vi "RX OOB Test Cases.vi"() -> (0 "error out":errorcluster, 2 "status":string, 3 "pass":bool)   [LabVIEW 2021]
uses:
  OOB_Rx/ChanMngOOB_Rx.lvclass/ChanMngOOB_Rx.ctl
  <vilib>/CIF Foundation/CIF Out of Band Commands/CIFOutOfBand.lvclass/CIFOutOfBand.ctl
  OOB_Rx/Typedef/OOB ChnMng Commands.ctl
  OOB_Rx/Typedef/Channel Connection Data.ctl
  OOB_Rx/Typedef/Channel Fault Data.ctl
  OOB_Rx/Typedef/FIFO Publisher.ctl
  <vilib>/CIF Foundation/CIF Channels Core/ChannelCommon/typedef/New FIFO Instance Configuration.ctl
  OOB_Rx/Private/Command Settings.vi
  <vilib>/CIF Foundation/CIF Out of Band Commands/Accessors/Write Local OOB Data.vi
  <vilib>/CIF Foundation/CIF Out of Band Commands/Accessors/Read Local OOB Data.vi
  <vilib>/CIF Foundation/CIF Out of Band Commands/Queue Command.vi
  <vilib>/CIF Foundation/CIF Out of Band Commands/Utilities/Command to Bitwise Command.vi
  <vilib>/CIF Foundation/CIF Out of Band Commands/Read Commands.vi
  OOB_Rx/Private/Read Payload.vi
  OOB_Rx/ChanMngOOB_Rx.lvclass
  C:/Program Files/National Instruments/LabVIEW 2021/vi.lib/CIF Foundation/CIF Out of Band Commands/CIFOutOfBand.lvclass
  <vilib>/CIF Foundation/CIF Out of Band Commands/Init OOB.vi
  <vilib>/CIF Foundation/CIF Out of Band Commands/CIFOutOfBand.lvclass
  <vilib>/CIF Foundation/CIF Channels Core/ChannelCommon/ChannelCommon.lvlib
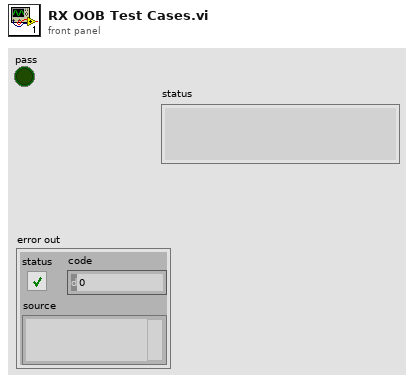
[diagram p1: front panel]
types:
  T1 = typedef "ChanMngOOB_Rx.lvclass/OOB ChnMng Commands.ctl" = enum8{"Connect Channel", "Force Channel", "Add FIFO Pub", "Remove FIFO Pub"}
  T2 = typedef "ChanMngOOB_Rx.lvclass/Channel Connection Data.ctl" = cluster{"Publisher Name":string, "Subscriber Name":string, "Connection Data":u8[]}
  T3 = typedef "ChanMngOOB_Rx.lvclass/Channel Fault Data.ctl" = cluster{"Channel Name":string, "Force Data":u8[], "Force Active":bool}
  T4 = typedef "ChanMngOOB_Rx.lvclass/FIFO Publisher.ctl" = cluster{"Publisher Name":string, "New FIFO Instance Config":T5}
  T5 = typedef "ChannelCommon.lvlib/New FIFO Instance Configuration.ctl" = cluster{"Primary":bool, "Backpressure":bool, "Message/FIFO Override":u32}
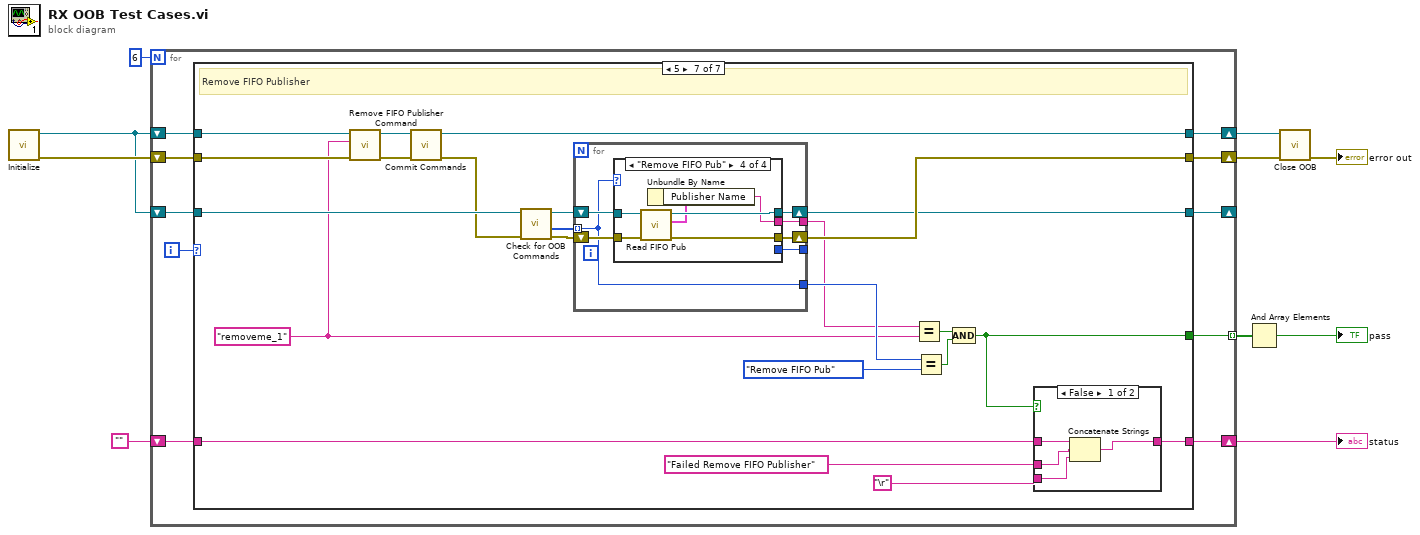
[diagram p0: block diagram]
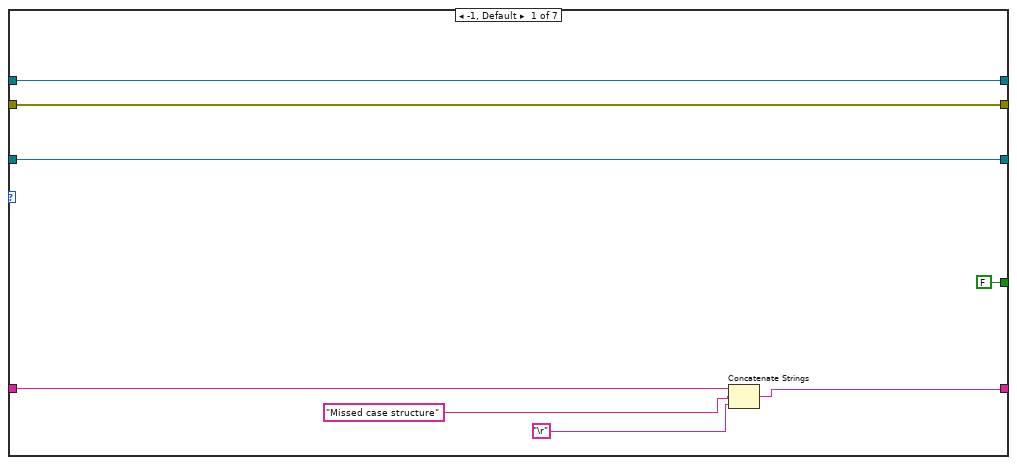
[diagram p2: hidden frame]
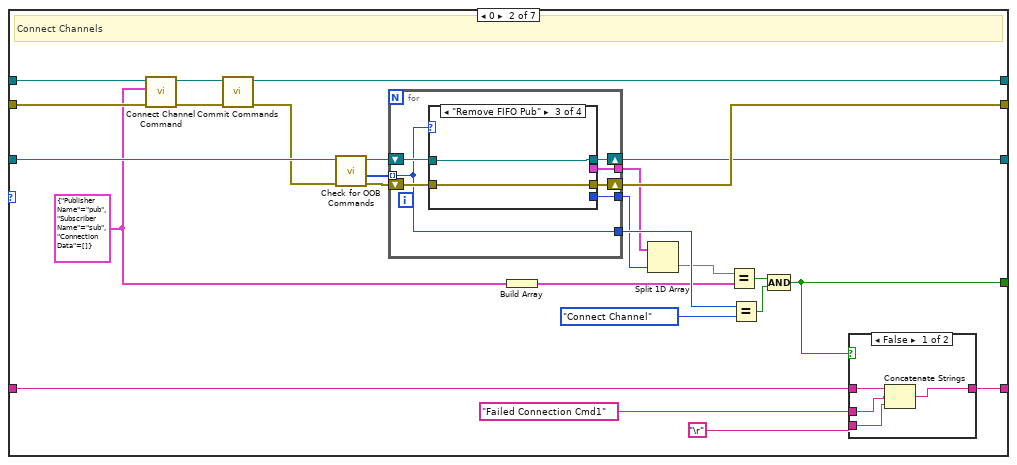
[diagram p3: hidden frame]
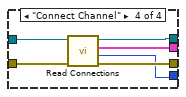
[diagram p6: hidden frame]
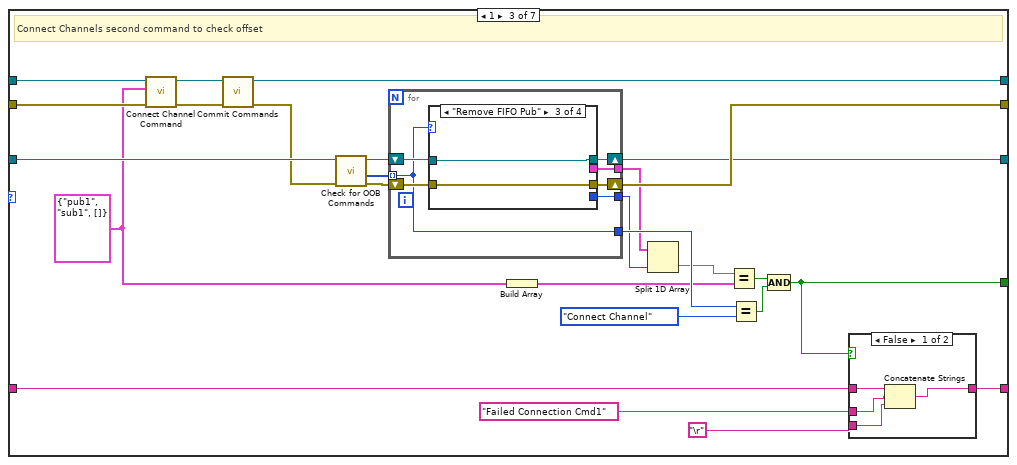
[diagram p8: hidden frame]
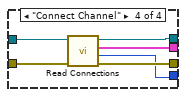
[diagram p11: hidden frame]
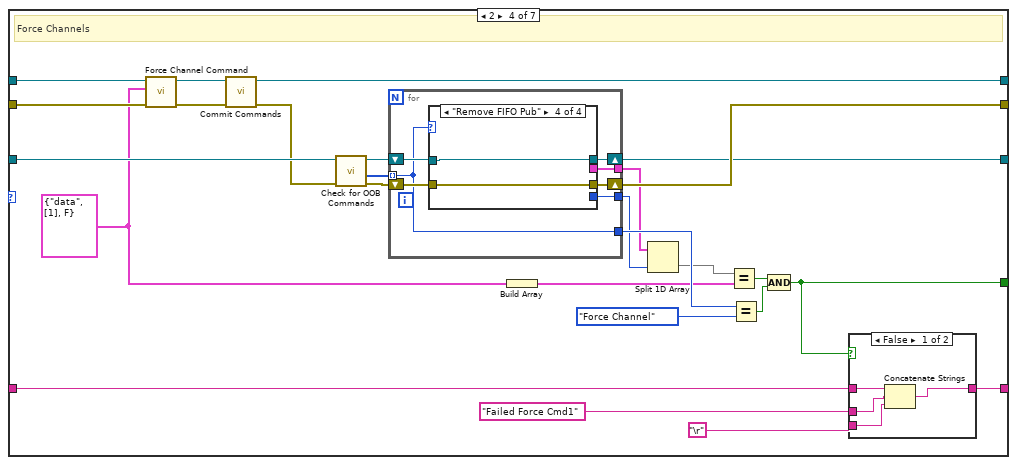
[diagram p13: hidden frame]
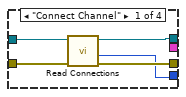
[diagram p14: hidden frame]
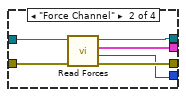
[diagram p15: hidden frame]
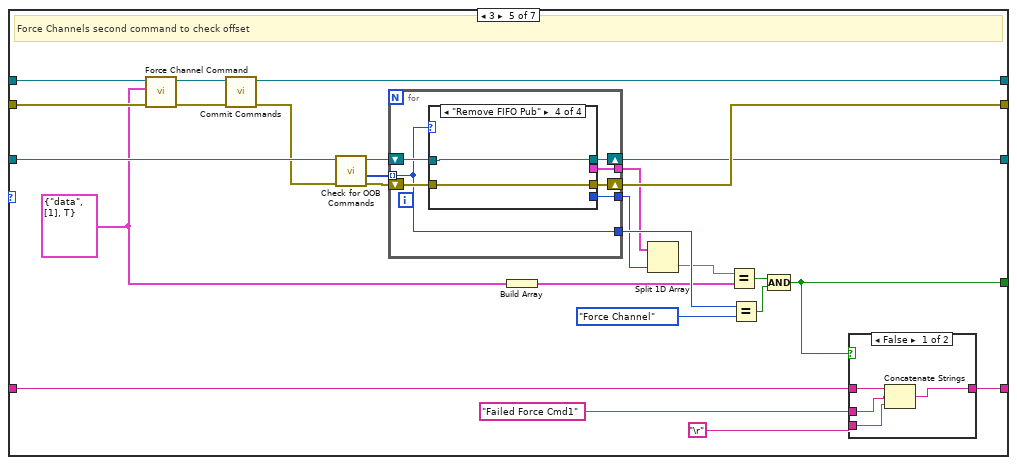
[diagram p18: hidden frame]
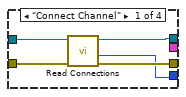
[diagram p19: hidden frame]
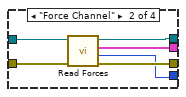
[diagram p20: hidden frame]
diagram:
  n1 = call "Initialize.vi"() -> ("error out"=w2:errorcluster, "CoreOOB_Rx out"=w1:refnum<class "ChanMngOOB_Rx.lvclass">)  [unwired: 10 in]
  n2 = for {
    N: 6 -> [_]
    tunnel: [w20] -> w8 mode=indexing
    shift-right: [w17] -> w9
    shift-left: w2 -> [w19]
    shift-right: [w15] -> w10
    shift-left: w1 -> [w18]
    shift-right: [w13] -> _
    shift-left: w1 -> [w14]
    shift-right: [w11] -> w5
    shift-left: "" -> [w12]
    i -> [w16]
    n3 = case shown="5" w16 {
      tunnel: [FALSE w33 w83 w135 w188 w243 w295] -> w20
      tunnel: w19 -> [w26 w41 w91 w141 w194 w238 w289]
      tunnel: w18 -> [w28 w42 w92 w142 w195 w240 w291]
      tunnel: [w26 w54 w104 w154 w207 w257 w309] -> w17
      tunnel: [w28 w29 w79 w129 w182 w241 w293] -> w15
      tunnel: w14 -> [w27 w48 w98 w148 w201 w251 w303]
      tunnel: [w27 w53 w103 w153 w206 w256 w308] -> w13
      tunnel: w12 -> [w23 w52 w102 w152 w205 w255 w307]
      tunnel: [w22 w51 w101 w151 w204 w254 w306] -> w11
      frame -1, Default {
        n4 = Concatenate Strings(w23, "Missed case structure", "\r") -> (w22:string)
      }
      frame 0 {
        w37 = T2 {"Publisher Name"="pub", "Subscriber Name"="sub", "Connection Data"=[]} ("Channel Connection Data")
        # "Connect Channels"
        n5 = call "Connect Channel Command.vi"("error in"=w41, "Channel Connection Data"=w37, "CoreOOB_Rx in"=w42) -> ("error out"=w31:errorcluster, "CoreOOB_Rx out"=w32:refnum<class "ChanMngOOB_Rx.lvclass">)  [unwired: 7 in]
        n6 = call <vilib>:"Commit Commands.vi"("error in"=w31, "OOB in"=w32) -> ("error out"=w30:errorcluster, "OOB out"=w29:refnum<class "ChanMngOOB_Rx.lvclass">)  [unwired: 8 in]
        n7 = call "Check for OOB Commands.vi"("error in (no error)"=w30, "CoreOOB_Rx in"=w48) -> ("error out"=w47:errorcluster, "Commands"=w45:T1[], "CoreOOB_Rx out"=w46:refnum<class "ChanMngOOB_Rx.lvclass">)  [unwired: 6 in, 1 out]
        n8 = for {
          tunnel: w45 -> [w57] mode=indexing
          shift-right: [w61] -> w54
          shift-left: w47 -> [w59]
          shift-right: [w60] -> w53
          shift-left: w46 -> [w58]
          tunnel: [w57] -> w44
          tunnel: [w56] -> w40
          tunnel: [w55] -> w39
          n9 = case shown="\"Remove FIFO Pub\"" w57 {
            tunnel: w58 -> [w63 w65 w67 w73]
            tunnel: w59 -> [w62 w64 w66 w72]
            tunnel: [w63 w65 w67 w71] -> w60
            tunnel: [w62 w64 w66 w70] -> w61
            tunnel: [_ _ _ w69] -> w56
            tunnel: [_ _ _ w68] -> w55
            frame "Force Channel" {
            }
            frame "Add FIFO Pub" {
            }
            frame "Remove FIFO Pub" {
            }
            frame "Connect Channel" {
              n10 = call "Read Connections.vi"("error in"=w72, "CoreOOB_Rx in"=w73) -> ("error out"=w70:errorcluster, "Offset"=w68:i32, "Connections"=w69:T2[], "CoreOOB_Rx out"=w71:refnum<class "ChanMngOOB_Rx.lvclass">)  [unwired: 6 in]
            }
          }
        }
        n11 = Build Array(w37) -> (w36:T2[])
        n12 = Split 1D Array(array=w40, index=w39) -> (second subarray=w38:T2[])  [unwired: 1 out]
        n13 = Equal?(x=w38, y=w36) -> (x = y?=w35:bool)
        n14 = Equal?(x=w44, y=OOB_ChnMng_Commands."Connect Channel") -> (x = y?=w34:bool)
        n15 = Compound Arithmetic op=AND(w35, w34) -> (w33:bool)
        n16 = case shown="False" w33 {
          tunnel: w52 -> [w77 w78]
          tunnel: [w74 w78] -> w51
          tunnel: "Failed Connection Cmd1" -> [w76 _]
          tunnel: "\r" -> [w75 _]
          frame False {
            n17 = Concatenate Strings(w77, w76, w75) -> (w74:string)
          }
          frame True {
          }
        }
      }
      frame 1 {
        w87 = T2 {"Publisher Name"="pub1", "Subscriber Name"="sub1", "Connection Data"=[]} ("Channel Connection Data")
        # "Connect Channels second command to check offset"
        n18 = call "Connect Channel Command.vi"("error in"=w91, "Channel Connection Data"=w87, "CoreOOB_Rx in"=w92) -> ("error out"=w81:errorcluster, "CoreOOB_Rx out"=w82:refnum<class "ChanMngOOB_Rx.lvclass">)  [unwired: 7 in]
        n19 = call <vilib>:"Commit Commands.vi"("error in"=w81, "OOB in"=w82) -> ("error out"=w80:errorcluster, "OOB out"=w79:refnum<class "ChanMngOOB_Rx.lvclass">)  [unwired: 8 in]
        n20 = call "Check for OOB Commands.vi"("error in (no error)"=w80, "CoreOOB_Rx in"=w98) -> ("error out"=w97:errorcluster, "Commands"=w95:T1[], "CoreOOB_Rx out"=w96:refnum<class "ChanMngOOB_Rx.lvclass">)  [unwired: 6 in, 1 out]
        n21 = for {
          tunnel: w95 -> [w107] mode=indexing
          shift-right: [w111] -> w104
          shift-left: w97 -> [w109]
          shift-right: [w110] -> w103
          shift-left: w96 -> [w108]
          tunnel: [w107] -> w94
          tunnel: [w106] -> w90
          tunnel: [w105] -> w89
          n22 = case shown="\"Remove FIFO Pub\"" w107 {
            tunnel: w108 -> [w113 w115 w117 w123]
            tunnel: w109 -> [w112 w114 w116 w122]
            tunnel: [w113 w115 w117 w121] -> w110
            tunnel: [w112 w114 w116 w120] -> w111
            tunnel: [_ _ _ w119] -> w106
            tunnel: [_ _ _ w118] -> w105
            frame "Force Channel" {
            }
            frame "Add FIFO Pub" {
            }
            frame "Remove FIFO Pub" {
            }
            frame "Connect Channel" {
              n23 = call "Read Connections.vi"("error in"=w122, "CoreOOB_Rx in"=w123) -> ("error out"=w120:errorcluster, "Offset"=w118:i32, "Connections"=w119:T2[], "CoreOOB_Rx out"=w121:refnum<class "ChanMngOOB_Rx.lvclass">)  [unwired: 6 in]
            }
          }
        }
        n24 = Build Array(w87) -> (w86:T2[])
        n25 = Split 1D Array(array=w90, index=w89) -> (second subarray=w88:T2[])  [unwired: 1 out]
        n26 = Equal?(x=w88, y=w86) -> (x = y?=w85:bool)
        n27 = Equal?(x=w94, y=OOB_ChnMng_Commands."Connect Channel") -> (x = y?=w84:bool)
        n28 = Compound Arithmetic op=AND(w85, w84) -> (w83:bool)
        n29 = case shown="False" w83 {
          tunnel: w102 -> [w127 w128]
          tunnel: [w124 w128] -> w101
          tunnel: "Failed Connection Cmd1" -> [w126 _]
          tunnel: "\r" -> [w125 _]
          frame False {
            n30 = Concatenate Strings(w127, w126, w125) -> (w124:string)
          }
          frame True {
          }
        }
      }
      frame 2 {
        w134 = T3 {"Channel Name"="data", "Force Data"=[1], "Force Active"=FALSE} ("Channel Force Data")
        # "Force Channels"
        n31 = call "Force Channel Command.vi"("error in"=w141, "Channel Force Data"=w134, "CoreOOB_Rx in"=w142) -> ("error out"=w131:errorcluster, "CoreOOB_Rx out"=w132:refnum<class "ChanMngOOB_Rx.lvclass">)  [unwired: 7 in]
        n32 = call <vilib>:"Commit Commands.vi"("error in"=w131, "OOB in"=w132) -> ("error out"=w130:errorcluster, "OOB out"=w129:refnum<class "ChanMngOOB_Rx.lvclass">)  [unwired: 8 in]
        n33 = call "Check for OOB Commands.vi"("error in (no error)"=w130, "CoreOOB_Rx in"=w148) -> ("error out"=w147:errorcluster, "Commands"=w145:T1[], "CoreOOB_Rx out"=w146:refnum<class "ChanMngOOB_Rx.lvclass">)  [unwired: 6 in, 1 out]
        n34 = for {
          tunnel: w145 -> [w157] mode=indexing
          shift-right: [w161] -> w154
          shift-left: w147 -> [w159]
          shift-right: [w160] -> w153
          shift-left: w146 -> [w158]
          tunnel: [w157] -> w144
          tunnel: [w156] -> w140
          tunnel: [w155] -> w139
          n35 = case shown="\"Remove FIFO Pub\"" w157 {
            tunnel: w158 -> [w166 w172 w174 w176]
            tunnel: w159 -> [w165 w171 w173 w175]
            tunnel: [w164 w170 w174 w176] -> w160
            tunnel: [w163 w169 w173 w175] -> w161
            tunnel: [_ w168 _ _] -> w156
            tunnel: [w162 w167 _ _] -> w155
            frame "Connect Channel" {
              n36 = call "Read Connections.vi"("error in"=w165, "CoreOOB_Rx in"=w166) -> ("error out"=w163:errorcluster, "Offset"=w162:i32, "CoreOOB_Rx out"=w164:refnum<class "ChanMngOOB_Rx.lvclass">)  [unwired: 6 in, 1 out]
            }
            frame "Force Channel" {
              n37 = call "Read Forces.vi"("error in"=w171, "CoreOOB_Rx in"=w172) -> ("error out"=w169:errorcluster, "Offset"=w167:i32, "Forces"=w168:T3[], "CoreOOB_Rx out"=w170:refnum<class "ChanMngOOB_Rx.lvclass">)  [unwired: 6 in]
            }
            frame "Add FIFO Pub" {
            }
            frame "Remove FIFO Pub" {
            }
          }
        }
        n38 = Build Array(w134) -> (w133:T3[])
        n39 = Split 1D Array(array=w140, index=w139) -> (second subarray=w138:T3[])  [unwired: 1 out]
        n40 = Equal?(x=w138, y=w133) -> (x = y?=w137:bool)
        n41 = Equal?(x=w144, y=OOB_ChnMng_Commands."Force Channel") -> (x = y?=w136:bool)
        n42 = Compound Arithmetic op=AND(w137, w136) -> (w135:bool)
        n43 = case shown="False" w135 {
          tunnel: w152 -> [w180 w181]
          tunnel: [w177 w181] -> w151
          tunnel: "Failed Force Cmd1" -> [w179 _]
          tunnel: "\r" -> [w178 _]
          frame False {
            n44 = Concatenate Strings(w180, w179, w178) -> (w177:string)
          }
          frame True {
          }
        }
      }
      frame 3 {
        w187 = T3 {"Channel Name"="data", "Force Data"=[1], "Force Active"=TRUE} ("Channel Force Data")
        # "Force Channels second command to check offset"
        n45 = call "Force Channel Command.vi"("error in"=w194, "Channel Force Data"=w187, "CoreOOB_Rx in"=w195) -> ("error out"=w184:errorcluster, "CoreOOB_Rx out"=w185:refnum<class "ChanMngOOB_Rx.lvclass">)  [unwired: 7 in]
        n46 = call <vilib>:"Commit Commands.vi"("error in"=w184, "OOB in"=w185) -> ("error out"=w183:errorcluster, "OOB out"=w182:refnum<class "ChanMngOOB_Rx.lvclass">)  [unwired: 8 in]
        n47 = call "Check for OOB Commands.vi"("error in (no error)"=w183, "CoreOOB_Rx in"=w201) -> ("error out"=w200:errorcluster, "Commands"=w198:T1[], "CoreOOB_Rx out"=w199:refnum<class "ChanMngOOB_Rx.lvclass">)  [unwired: 6 in, 1 out]
        n48 = for {
          tunnel: w198 -> [w210] mode=indexing
          shift-right: [w214] -> w207
          shift-left: w200 -> [w212]
          shift-right: [w213] -> w206
          shift-left: w199 -> [w211]
          tunnel: [w210] -> w197
          tunnel: [w209] -> w193
          tunnel: [w208] -> w192
          n49 = case shown="\"Remove FIFO Pub\"" w210 {
            tunnel: w211 -> [w219 w225 w227 w229]
            tunnel: w212 -> [w218 w224 w226 w228]
            tunnel: [w217 w223 w227 w229] -> w213
            tunnel: [w216 w222 w226 w228] -> w214
            tunnel: [_ w221 _ _] -> w209
            tunnel: [w215 w220 _ _] -> w208
            frame "Connect Channel" {
              n50 = call "Read Connections.vi"("error in"=w218, "CoreOOB_Rx in"=w219) -> ("error out"=w216:errorcluster, "Offset"=w215:i32, "CoreOOB_Rx out"=w217:refnum<class "ChanMngOOB_Rx.lvclass">)  [unwired: 6 in, 1 out]
            }
            frame "Force Channel" {
              n51 = call "Read Forces.vi"("error in"=w224, "CoreOOB_Rx in"=w225) -> ("error out"=w222:errorcluster, "Offset"=w220:i32, "Forces"=w221:T3[], "CoreOOB_Rx out"=w223:refnum<class "ChanMngOOB_Rx.lvclass">)  [unwired: 6 in]
            }
            frame "Add FIFO Pub" {
            }
            frame "Remove FIFO Pub" {
            }
          }
        }
        n52 = Build Array(w187) -> (w186:T3[])
        n53 = Split 1D Array(array=w193, index=w192) -> (second subarray=w191:T3[])  [unwired: 1 out]
        n54 = Equal?(x=w191, y=w186) -> (x = y?=w190:bool)
        n55 = Equal?(x=w197, y=OOB_ChnMng_Commands."Force Channel") -> (x = y?=w189:bool)
        n56 = Compound Arithmetic op=AND(w190, w189) -> (w188:bool)
        n57 = case shown="False" w188 {
          tunnel: w205 -> [w233 w234]
          tunnel: [w230 w234] -> w204
          tunnel: "Failed Force Cmd1" -> [w232 _]
          tunnel: "\r" -> [w231 _]
          frame False {
            n58 = Concatenate Strings(w233, w232, w231) -> (w230:string)
          }
          frame True {
          }
        }
      }
      frame 4 {
        w236 = T4 {"Publisher Name"="pubme", "New FIFO Instance Config"={"Primary"=TRUE, "Backpressure"=FALSE, "Message/FIFO Override"=500}} ("New FIFO Pub")
        # "Add FIFO Publisher"
        n59 = call "Add FIFO Publisher Command.vi"("error in"=w238, "New FIFO Pub"=w236, "CoreOOB_Rx in"=w240) -> ("error out"=w237:errorcluster, "CoreOOB_Rx out"=w239:refnum<class "ChanMngOOB_Rx.lvclass">)  [unwired: 7 in]
        n60 = call <vilib>:"Commit Commands.vi"("error in"=w237, "OOB in"=w239) -> ("error out"=w242:errorcluster, "OOB out"=w241:refnum<class "ChanMngOOB_Rx.lvclass">)  [unwired: 8 in]
        n61 = call "Check for OOB Commands.vi"("error in (no error)"=w242, "CoreOOB_Rx in"=w251) -> ("error out"=w250:errorcluster, "Commands"=w248:T1[], "CoreOOB_Rx out"=w249:refnum<class "ChanMngOOB_Rx.lvclass">)  [unwired: 6 in, 1 out]
        n62 = for {
          tunnel: w248 -> [w260] mode=indexing
          shift-right: [w264] -> w257
          shift-left: w250 -> [w262]
          shift-right: [w263] -> w256
          shift-left: w249 -> [w261]
          tunnel: [w260] -> w247
          tunnel: [w259] -> w235
          tunnel: [w258] -> _
          n63 = case shown="\"Add FIFO Pub\"" w260 {
            tunnel: w261 -> [w269 w274 w279 w281]
            tunnel: w262 -> [w268 w273 w278 w280]
            tunnel: [w267 w272 w277 w281] -> w263
            tunnel: [w266 w271 w275 w280] -> w264
            tunnel: [_ _ w276 _] -> w259
            tunnel: [w265 w270 _ _] -> w258
            frame "Connect Channel" {
              n64 = call "Read Connections.vi"("error in"=w268, "CoreOOB_Rx in"=w269) -> ("error out"=w266:errorcluster, "Offset"=w265:i32, "CoreOOB_Rx out"=w267:refnum<class "ChanMngOOB_Rx.lvclass">)  [unwired: 6 in, 1 out]
            }
            frame "Force Channel" {
              n65 = call "Read Forces.vi"("error in"=w273, "CoreOOB_Rx in"=w274) -> ("error out"=w271:errorcluster, "Offset"=w270:i32, "CoreOOB_Rx out"=w272:refnum<class "ChanMngOOB_Rx.lvclass">)  [unwired: 6 in, 1 out]
            }
            frame "Add FIFO Pub" {
              n66 = call "Read FIFO Pub.vi"("error in"=w278, "CoreOOB_Rx in"=w279) -> ("error out"=w275:errorcluster, "FIFO Pub"=w276:T4, "CoreOOB_Rx out"=w277:refnum<class "ChanMngOOB_Rx.lvclass">)  [unwired: 7 in]
            }
            frame "Remove FIFO Pub" {
            }
          }
        }
        n67 = Equal?(x=w235, y=w236) -> (x = y?=w245:bool)
        n68 = Equal?(x=w247, y=OOB_ChnMng_Commands."Add FIFO Pub") -> (x = y?=w244:bool)
        n69 = Compound Arithmetic op=AND(w245, w244) -> (w243:bool)
        n70 = case shown="False" w243 {
          tunnel: w255 -> [w285 w286]
          tunnel: [w282 w286] -> w254
          tunnel: "Failed Add FIFO Publisher" -> [w284 _]
          tunnel: "\r" -> [w283 _]
          frame False {
            n71 = Concatenate Strings(w285, w284, w283) -> (w282:string)
          }
          frame True {
          }
        }
      }
      frame 5 {
        w287 = "removeme_1" ("Publisher Name")
        # "Remove FIFO Publisher"
        n72 = call "Remove FIFO Publisher Command.vi"("error in"=w289, "Publisher Name"=w287, "CoreOOB_Rx in"=w291) -> ("error out"=w288:errorcluster, "CoreOOB_Rx out"=w290:refnum<class "ChanMngOOB_Rx.lvclass">)  [unwired: 7 in]
        n73 = call <vilib>:"Commit Commands.vi"("error in"=w288, "OOB in"=w290) -> ("error out"=w294:errorcluster, "OOB out"=w293:refnum<class "ChanMngOOB_Rx.lvclass">)  [unwired: 8 in]
        n74 = call "Check for OOB Commands.vi"("error in (no error)"=w294, "CoreOOB_Rx in"=w303) -> ("error out"=w302:errorcluster, "Commands"=w300:T1[], "CoreOOB_Rx out"=w301:refnum<class "ChanMngOOB_Rx.lvclass">)  [unwired: 6 in, 1 out]
        n75 = for {
          tunnel: w300 -> [w312] mode=indexing
          shift-right: [w316] -> w309
          shift-left: w302 -> [w314]
          shift-right: [w315] -> w308
          shift-left: w301 -> [w313]
          tunnel: [w312] -> w299
          tunnel: [w311] -> w292
          tunnel: [w310] -> _
          n76 = case shown="\"Remove FIFO Pub\"" w312 {
            tunnel: w313 -> [w321 w326 w330 w336]
            tunnel: w314 -> [w320 w325 w329 w335]
            tunnel: [w319 w324 w328 w334] -> w315
            tunnel: [w318 w323 w327 w333] -> w316
            tunnel: [_ _ _ w331] -> w311
            tunnel: [w317 w322 _ _] -> w310
            frame "Connect Channel" {
              n77 = call "Read Connections.vi"("error in"=w320, "CoreOOB_Rx in"=w321) -> ("error out"=w318:errorcluster, "Offset"=w317:i32, "CoreOOB_Rx out"=w319:refnum<class "ChanMngOOB_Rx.lvclass">)  [unwired: 6 in, 1 out]
            }
            frame "Force Channel" {
              n78 = call "Read Forces.vi"("error in"=w325, "CoreOOB_Rx in"=w326) -> ("error out"=w323:errorcluster, "Offset"=w322:i32, "CoreOOB_Rx out"=w324:refnum<class "ChanMngOOB_Rx.lvclass">)  [unwired: 6 in, 1 out]
            }
            frame "Add FIFO Pub" {
              n79 = call "Read FIFO Pub.vi"("error in"=w329, "CoreOOB_Rx in"=w330) -> ("error out"=w327:errorcluster, "CoreOOB_Rx out"=w328:refnum<class "ChanMngOOB_Rx.lvclass">)  [unwired: 7 in, 1 out]
            }
            frame "Remove FIFO Pub" {
              n80 = call "Read FIFO Pub.vi"("error in"=w335, "CoreOOB_Rx in"=w336) -> ("error out"=w333:errorcluster, "FIFO Pub"=w332:T4, "CoreOOB_Rx out"=w334:refnum<class "ChanMngOOB_Rx.lvclass">)  [unwired: 7 in]
              n81 = Unbundle By Name(w332) -> ("Publisher Name"=w331:string)
            }
          }
        }
        n82 = Equal?(x=w292, y=w287) -> (x = y?=w297:bool)
        n83 = Equal?(x=w299, y=OOB_ChnMng_Commands."Remove FIFO Pub") -> (x = y?=w296:bool)
        n84 = Compound Arithmetic op=AND(w297, w296) -> (w295:bool)
        n85 = case shown="False" w295 {
          tunnel: w307 -> [w340 w341]
          tunnel: [w337 w341] -> w306
          tunnel: "Failed Remove FIFO Publisher" -> [w339 _]
          tunnel: "\r" -> [w338 _]
          frame False {
            n86 = Concatenate Strings(w340, w339, w338) -> (w337:string)
          }
          frame True {
          }
        }
      }
    }
  }
  "status" <- w5
  n87 = And Array Elements(Boolean array=w8) -> (logical AND=→"pass":bool)
  n88 = call <vilib>:"Close OOB.vi"("error in"=w9, "OOB in"=w10) -> ("error out"=→"error out":errorcluster)  [unwired: 9 in]
